vi "Configure Measurement.vi"(7 "range (-1.0: Auto)":dbl=-1.0 format="%^.2e", 8 "error in (no error)":errorcluster, 9 "absolute resolution (0.001)":dbl=0.001 format="%^.2e", 10 "measurement function (DC Volts)":i32(ring)=1 items=["DC Volts"=1, "AC Volts"=2, "DC Current"=3, "AC Current"=4, "2 Wire Resistance"=5, "4 Wire Resistance"=101, "AC + DC Volts"=106, "AC + DC Current"=107, "Frequency"=104, "Period"=105, "Temperature"=108], 11 "CS++DMM in":refnum<class "CS++DMM.lvclass">) -> (0 "error out":errorcluster, 3 "CS++DMM out":refnum<class "CS++DMM.lvclass">)   [LabVIEW 2013, in "CS++DMM.lvlib" / "CS++DMM.lvclass"]
doc: "This VI configures the common properties of the DMM. These properties include the measurement function, maximum range, and resolution."
uses:
  CS++DMM.lvclass
  CSPP_Core/Classes/CS++ProcessVariables/ProcessVariable/PV.lvclass
  CS++DMM.lvclass/CS++DMM.ctl
  CSPP_Core/Classes/CS++ProcessVariables/PVConnection/PVConnection.lvclass
  CSPP_Core/Classes/CS++ProcessVariables/ProcessVariable/PV.lvclass/PV.ctl
  CSPP_Core/Classes/CS++ProcessVariables/ProcessVariable/Write Data.vi
  CSPP_Core/Classes/CS++ProcessVariables/ProcessVariable/Write Timestamp.vi
  CSPP_Core/Classes/CS++ProcessVariables/ProcessVariable/Write Quality.vi
  CSPP_Core/Classes/CS++ProcessVariables/ProcessVariable/Write status.vi
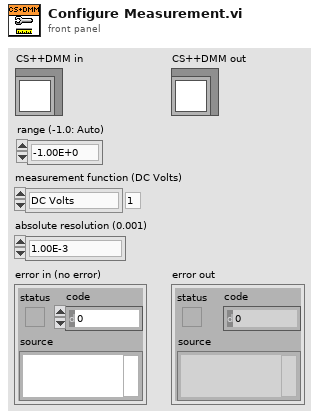
[diagram p1: front panel]
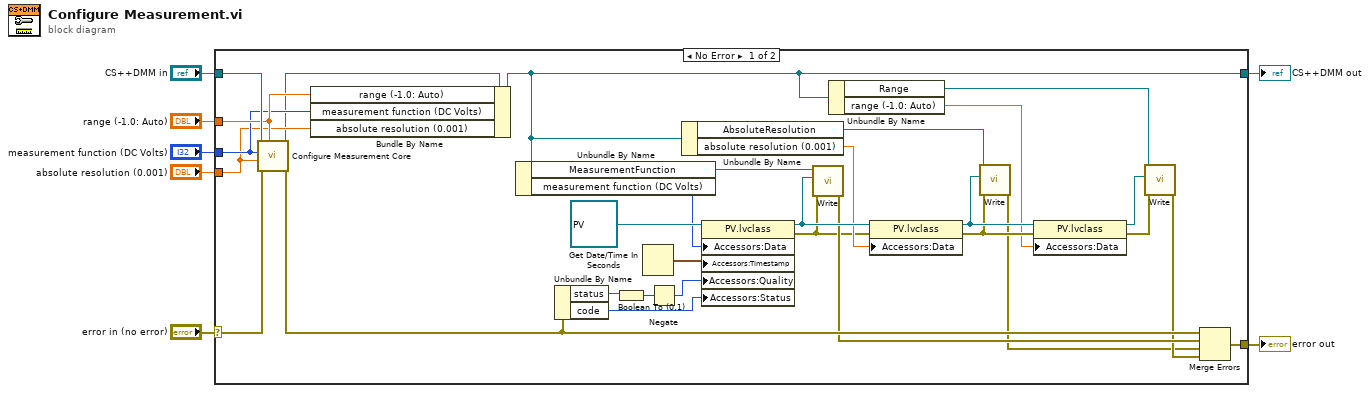
[diagram p0: block diagram]
diagram:
  n1 = case shown="No Error" "error in (no error)" {
    selector: "error in (no error)" -> [w36 w39]
    tunnel: [w19 w39] -> w6
    tunnel: [w16 w38] -> w4
    tunnel: "CS++DMM in" -> [w37 w38]
    tunnel: "range (-1.0: Auto)" -> [w35 _]
    tunnel: "measurement function (DC Volts)" -> [w34 _]
    tunnel: "absolute resolution (0.001)" -> [w33 _]
    frame No Error {
      n2 = call-dynamic "Configure Measurement Core.vi"("range (-1.0: Auto)"=w35, "error in (no error)"=w36, "absolute resolution (0.001)"=w33, "measurement function (DC Volts)"=w34, "CS++DMM in"=w37) -> ("error out"=w23:errorcluster, "CS++DMM out"=w32:refnum<class "CS++DMM.lvclass">)  [unwired: 5 in]
      n3 = Bundle By Name(cluster=w32, "range (-1.0: Auto)"=w35, "measurement function (DC Volts)"=w34, "absolute resolution (0.001)"=w33) -> (w16:refnum<class "CS++DMM.lvclass">)
      n4 = Unbundle By Name(w16) -> ("MeasurementFunction"=w31:refnum<class "PVConnection.lvclass">, "measurement function (DC Volts)"=w29:i32)
      n5 = Unbundle By Name(w23) -> ("status"=w28:bool, "code"=w25:i32)
      n6 = Boolean To (0,1)(Boolean=w28) -> (0, 1=w27:i16)
      n7 = Get Date/Time In Seconds() -> (seconds since 1Jan1904=w24:timestamp)
      n8 = Negate(x=w27) -> (-x=w26:i16)
      n9 = Unbundle By Name(w16) -> ("AbsoluteResolution"=w20:refnum<class "PVConnection.lvclass">, "absolute resolution (0.001)"=w21:dbl)
      n10 = property class="PV.lvclass"(reference=refnum<class "PV.lvclass"> refnum ("CS++ProcessVariables.lvlib:PV.lvclass"), "Accessors:Data"=w29, "Accessors:Timestamp"=w24, "Accessors:Quality"=w26, "Accessors:Status"=w25) -> (reference out=w22:refnum<class "PV.lvclass">, error out=w17:errorcluster)  [unwired: 1 in]
      n11 = call-dynamic "Write.vi"("error in (no error)"=w17, "PV"=w22, "PVConnection in"=w31) -> ("error out"=w18:errorcluster)  [unwired: 7 in, 1 out]
      n12 = Unbundle By Name(w16) -> ("Range"=w10:refnum<class "PVConnection.lvclass">, "range (-1.0: Auto)"=w11:dbl)
      n13 = property class="PV.lvclass"(reference=w22, error in=w17, "Accessors:Data"=w21) -> (reference out=w13:refnum<class "PV.lvclass">, error out=w12:errorcluster)
      n14 = call-dynamic "Write.vi"("error in (no error)"=w12, "PV"=w13, "PVConnection in"=w20) -> ("error out"=w8:errorcluster)  [unwired: 7 in, 1 out]
      n15 = property class="PV.lvclass"(reference=w13, error in=w12, "Accessors:Data"=w11) -> (reference out=w15:refnum<class "PV.lvclass">, error out=w14:errorcluster)
      n16 = call-dynamic "Write.vi"("error in (no error)"=w14, "PV"=w15, "PVConnection in"=w10) -> ("error out"=w9:errorcluster)  [unwired: 7 in, 1 out]
      n17 = Merge Errors(w23, w18, w8, w9) -> (w19:errorcluster)
    }
    frame Error {
    }
  }
  "error out" <- w6
  "CS++DMM out" <- w4
